vi "helperLoop.vi"(8 "error in (no error)":errorcluster, 11 "Actor wHelper in":refnum<class "Actor wHelper.lvclass">) -> (0 "error out":errorcluster, 3 "Actor wHelper out":refnum<class "Actor wHelper.lvclass">)   [LabVIEW 2017, in "Framework.lvlib" / "Actor wHelper.lvclass"]
uses:
  Actor wHelper.lvclass
  Actor wHelper.lvclass/Actor wHelper.ctl
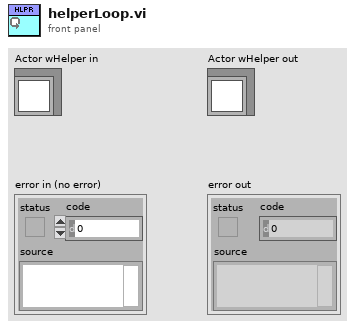
[diagram p1: front panel]
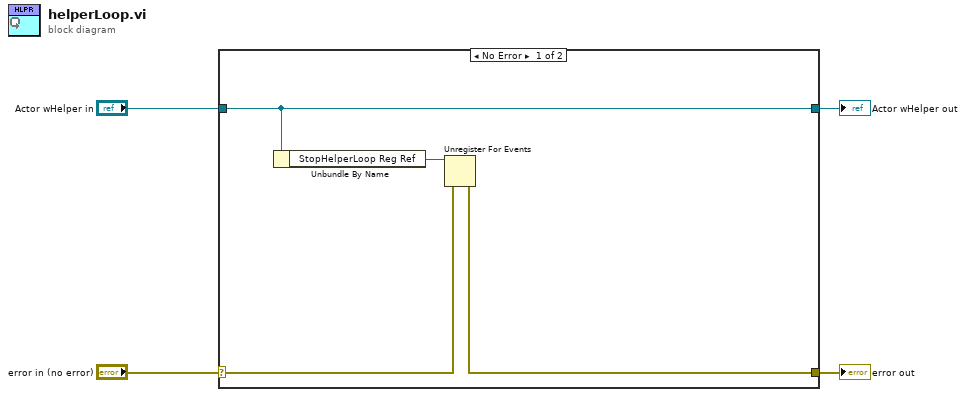
[diagram p0: block diagram]
diagram:
  n1 = case shown="No Error" "error in (no error)" {
    selector: "error in (no error)" -> [w6 w10]
    tunnel: [w5 w10] -> w3
    tunnel: [w8 w9] -> w1
    tunnel: "Actor wHelper in" -> [w8 w9]
    frame No Error {
      n2 = Unbundle By Name(w8) -> ("StopHelperLoop Reg Ref"=w7:refnum<event-registration>)
      n3 = Unregister For Events(event registration refnum=w7, error in=w6) -> (error out=w5:errorcluster)
    }
    frame Error {
    }
  }
  "error out" <- w3
  "Actor wHelper out" <- w1
